vi "Scan_For_Devices.vi"() -> (1 "Device Properties":string[][](array[string]))   [LabVIEW 2024]
uses:
  <vilib>/Analysis/1siggen.llb/Ramp Pattern by Delta.vi
  <vilib>/Analysis/NI_AALBase.lvlib
panel:
  in  "Number to Generate":u64=6
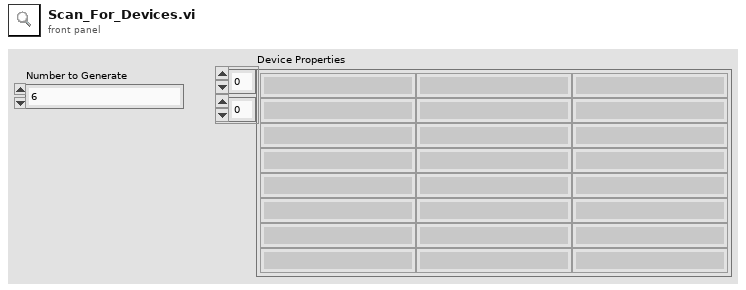
[diagram p1: front panel]
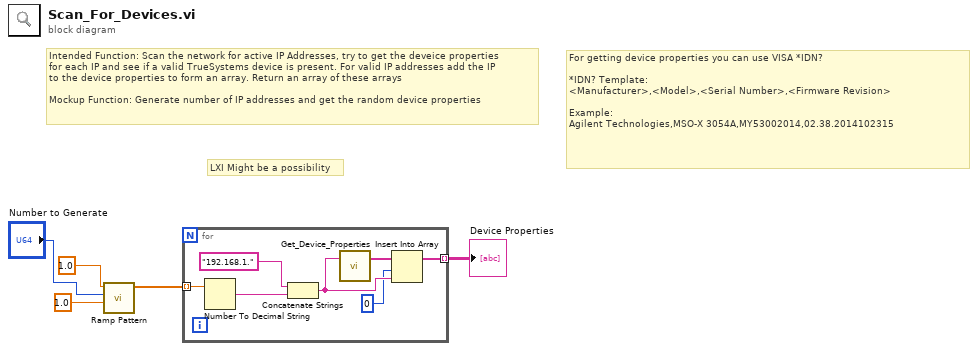
[diagram p0: block diagram]
diagram:
  # "LXI Might be a possibility"
  # "For getting device properties you can use VISA *IDN?\n\n*IDN? Template:\n<Manufacturer>,<Model>,<Serial Number>,<Firmware Revision>\n\nExample:\nAgilent Technologies,MSO-X 3054A,MY53002014,02.38.2014102315"
  # "Intended Function: Scan the network for active IP Addresses, try to get the deveice properties\nfor each IP and see if a valid TrueSystems device is present. For valid IP addresses add the IP\nto the device properties to form an array. Return an array of these arrays\n\nMockup Function: Generate number of IP addresses and get the random device properties"
  n1 = call-poly <vilib>:"Ramp Pattern.vi"("start"=1.0, "end"="Number to Generate", "delta"=1.0) -> ("Ramp Pattern"=w3:dbl[])  [unwired: 6 in, 2 out]
  n2 = for {
    tunnel: w3 -> [w7] mode=indexing
    tunnel: [w6] -> w2 mode=indexing
    n3 = Number To Decimal String(number=w7) -> (decimal integer string=w12:string)  [unwired: 1 in]
    n4 = Concatenate Strings("192.168.1.", w12) -> (w9:string)
    n5 = call "Get_Device_Properties.vi"("IP Address"=w9) -> ("Device Properties"=w10:string[])  [unwired: 2 in]
    n6 = Insert Into Array(array=w10, index=0, new element=w9) -> (w6:string[])
  }
  "Device Properties" <- w2
